vi "setState.vi"(8 "error in (no error)":errorcluster, 10 "State":cluster{"Value":i32, "Options":i32[]}[][](array[cluster]), 11 "SudukuState in":refnum<class "SudokuState.lvclass">) -> (0 "error out":errorcluster, 3 "SudukuState out":refnum<class "SudokuState.lvclass">)   [LabVIEW 2013, in "SudokuState.lvclass"]
uses:
  SudokuState.lvclass
  SudokuState.lvclass/SudokuState.ctl
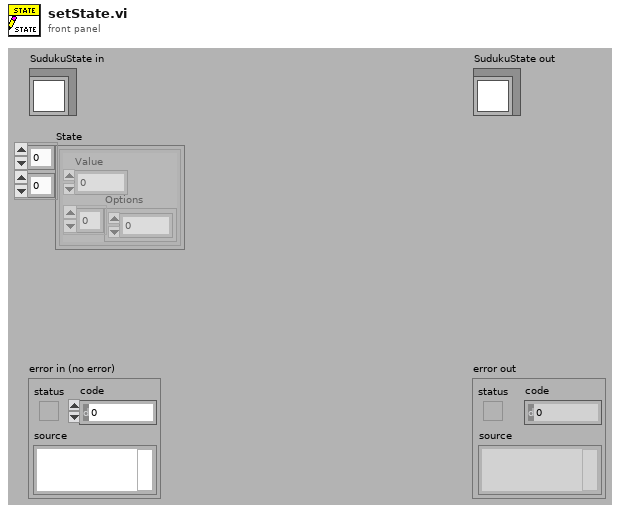
[diagram p1: front panel]
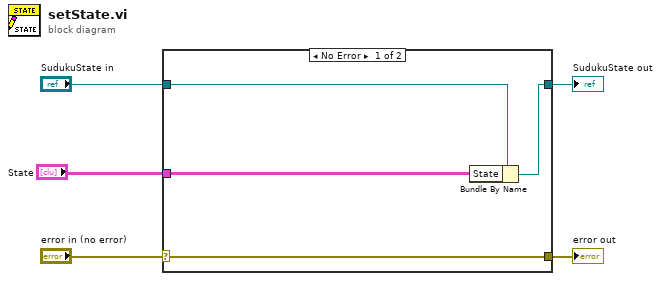
[diagram p0: block diagram]
diagram:
  n1 = case shown="No Error" "error in (no error)" {
    selector: "error in (no error)" -> [w9 w10]
    tunnel: [w9 w10] -> w4
    tunnel: [w7 w11] -> w2
    tunnel: "SudukuState in" -> [w8 w11]
    tunnel: "State" -> [w6 _]
    frame No Error {
      n2 = Bundle By Name(cluster=w8, "State"=w6) -> (w7:refnum<class "SudokuState.lvclass">)
    }
    frame Error {
    }
  }
  "error out" <- w4
  "SudukuState out" <- w2
